vi "Remove VI From Subpanel.vi"(8 "error in (no error)":errorcluster, 10 "subpanel VI":T1, 11 "VI Panel Layout in":refnum<class "VI Panel Layout.lvclass">) -> (0 "error out":errorcluster, 3 "VI Panel Layout out":refnum<class "VI Panel Layout.lvclass">)   [LabVIEW 2012, in "NI_SE_Front Panel Layout.lvlib" / "VI Panel Layout.lvclass"]
uses:
  VI Panel Layout.lvclass
  Subpanel VI Pair.ctl
  VI Panel Layout.lvclass/VI Panel Layout.ctl
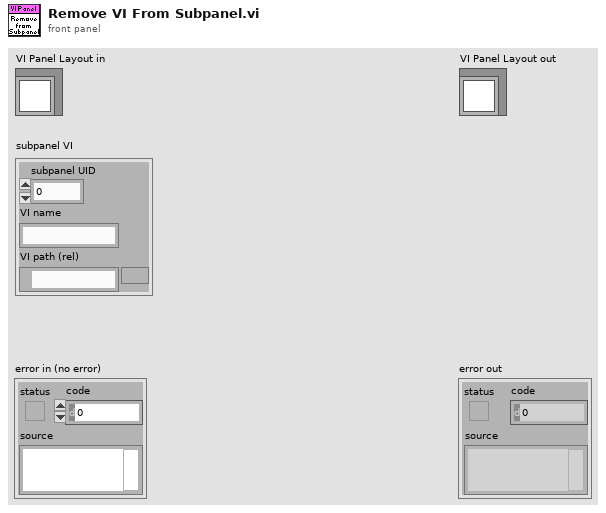
[diagram p1: front panel]
types:
  T1 = typedef "NI_SE_Front Panel Layout.lvlib/VI Panel Layout.lvclass/Subpanel VI Pair.ctl" = cluster{"subpanel UID":i32, "VI name":string, "VI path (rel)":path}
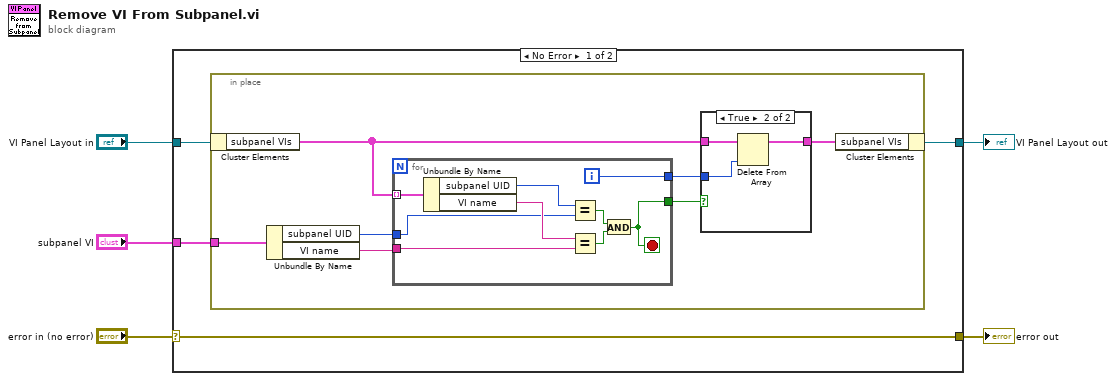
[diagram p0: block diagram]
diagram:
  n1 = case shown="No Error" "error in (no error)" {
    selector: "error in (no error)" -> [w9 w31]
    tunnel: [w9 w31] -> w4
    tunnel: [w6 w30] -> w2
    tunnel: "VI Panel Layout in" -> [w7 w30]
    tunnel: "subpanel VI" -> [w8 _]
    frame No Error {
      n2 = in-place {
        in-place-border: w8 -> [w16]
        n3 = in-place-cluster #1(w7) -> ("subpanel VIs"=w13:T1[])
        n4 = Unbundle By Name(w16) -> ("subpanel UID"=w15:i32, "VI name"=w14:string)
        n5 = for {
          tunnel: w13 -> [w29] mode=indexing
          tunnel: w14 -> [w28]
          tunnel: w15 -> [w25]
          tunnel: [w22] -> w11
          tunnel: [w21] -> w10
          i -> [w21]
          stop <- w22 stop-if-true
          n6 = Unbundle By Name(w29) -> ("subpanel UID"=w26:i32, "VI name"=w27:string)
          n7 = Equal?(x=w26, y=w25) -> (x = y?=w24:bool)
          n8 = Equal?(x=w27, y=w28) -> (x = y?=w23:bool)
          n9 = And(x=w24, y=w23) -> (x .and. y?=w22:bool)
        }
        n10 = case shown="True" w11 {
          tunnel: w13 -> [w17 w20]
          tunnel: [w17 w19] -> w12
          tunnel: w10 -> [_ w18]
          frame False {
          }
          frame True {
            n11 = Delete From Array(array=w20, index=w18) -> (array with subset deleted=w19:T1[])  [unwired: 1 in, 1 out]
          }
        }
        n12 = in-place-cluster #1("subpanel VIs"=w12) -> (w6:refnum<class "VI Panel Layout.lvclass">)
      }
    }
    frame Error {
    }
  }
  "error out" <- w4
  "VI Panel Layout out" <- w2
